vi "pp3b_DAQwriteDO.vi"(7 "Reset to zero":bool=TRUE, 8 "error in (no error)":errorcluster, 9 "Master-9 Digital":bool[](array[boolean]), 10 "Daq config":T1={"Sound AO"="Dev6/ao0", "Shock intesity AO"="Dev6/ao1", "Code_LED DO"="Dev6/port1:2", "Switch DI"="Dev6/port1/line0", "Webcam"="cam9", "Sound AO task"="", "Sound card task"=0, "Shock intensity AO task"="", "Code_LED DO task"="", "Switch DI task"="", "AO <=> Sound card"=FALSE, "Sound card"=0, "sample rate"=100000.0, "Variable shock"=TRUE, "Webcam on"=FALSE, "Waveform memo"={"t0"=timestamp(0 s since 1904-01-01), "dt"=1.0, "Y"=[]}, "First time"=FALSE, "Tone trigger"="", "Master-9 DO"="Dev6/port0/line5:7", "Master-9 DO task"=""} {"sample rate" min=8000.0; "Sound card task" format="%.0x"}, 11 "DAQ Digital In":u16 format="%b") -> (0 "error out":errorcluster)   [LabVIEW 2013]
uses:
  pp3b_CTL_DaqConfig.ctl
  <vilib>/userdefined/High Color/IMAQdx.ctl
  <vilib>/sound2/lvsound2.llb/Sound Output Task ID.ctl
  <vilib>/DAQmx/write.llb/DAQmx Write (Digital 1D U16 1Chan NSamp).vi
  <vilib>/DAQmx/write.llb/DAQmx Write (Digital 1D Bool 1Chan 1Samp).vi
  <vilib>/DAQmx/miscellaneous.llb/DAQmx Fill In Error Info.vi
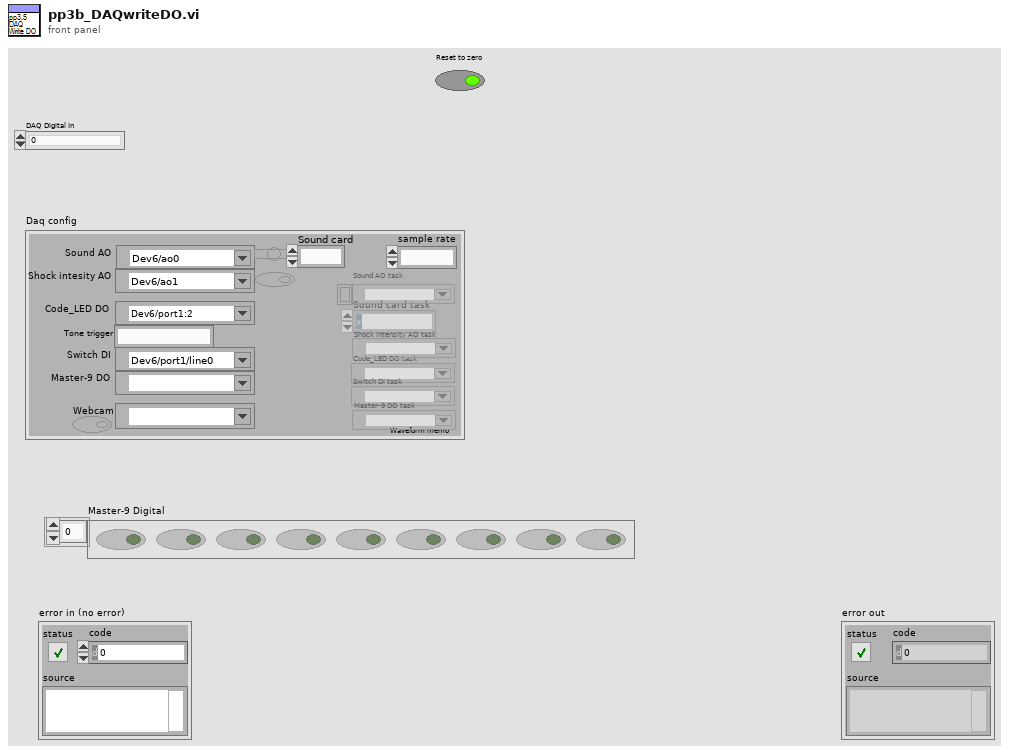
[diagram p1: front panel]
types:
  T1 = typedef "pp3b_CTL_DaqConfig.ctl" = cluster{"Sound AO":tag, "Shock intesity AO":tag, "Code_LED DO":tag, "Switch DI":tag, "Webcam":T2, "Sound AO task":refnum<k21>, "Sound card task":T3, "Shock intensity AO task":refnum<k21>, "Code_LED DO task":refnum<k21>, "Switch DI task":refnum<k21>, "AO <=> Sound card":bool, "Sound card":u32, "sample rate":dbl, "Variable shock":bool, "Webcam on":bool, "Waveform memo":waveform(dbl), "First time":bool, "Tone trigger":string, "Master-9 DO":tag, "Master-9 DO task":refnum<k21>}
  T2 = typedef "IMAQdx.ctl" = refnum<k21>
  T3 = typedef "Sound Output Task ID.ctl" = u32
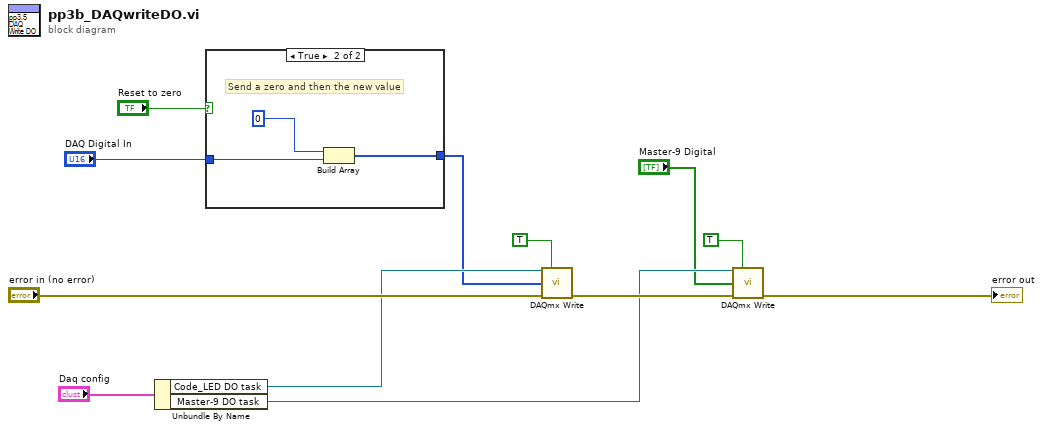
[diagram p0: block diagram]
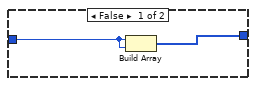
[diagram p2: hidden frame]
diagram:
  n1 = Unbundle By Name("Daq config") -> ("Code_LED DO task"=w10:refnum<k21>, "Master-9 DO task"=w2:refnum<k21>)
  n2 = case shown="True" "Reset to zero" {
    tunnel: "DAQ Digital In" -> [w13 w16]
    tunnel: [w14 w15] -> w6
    frame False {
      n3 = Build Array(w13, w13) -> (w14:u16[])
    }
    frame True {
      # "Send a zero and then the new value"
      n4 = Build Array(u16 0 ("Waveform"), w16) -> (w15:u16[])
    }
  }
  n5 = call-poly <vilib>:"DAQmx Write.vi"("task/channels in"=w10, "auto start"=TRUE, "data"=w6, "error in"="error in (no error)") -> ("error out"=w3:errorcluster)  [unwired: 9 in, 2 out]
  n6 = call-poly <vilib>:"DAQmx Write.vi"("task/channels in"=w2, "auto start"=TRUE, "data"="Master-9 Digital", "error in"=w3) -> ("error out"=→"error out":errorcluster)  [unwired: 9 in, 2 out]
